vi "ExSimpleAsyncExample.vi"() -> ()   [LabVIEW 2010]
panel:
  in  "Trigger Edge":u32(ring)=1 items=["N/A", "Positive (leading) edge", "Negative (falling) edge"]
  in  "Timing Mode":u32(ring)=1 items=["N/A", "Free Run/Timed", "Trigger First (PM only)", "Ext Sync/Strobed ", "Variable Exp (PM only)", "Flash Mode (PM only)"]
  in  "Temperature":dbl format="%.2f"
  in  "Exposure":dbl min=0.0 step=0.001 format="%.3f"
  in  "stop":bool
  in  "Store":bool
  out "error out":errorcluster
  in  "error in (no error)":errorcluster
  # "ExSimipleAsyncExample:\nThis is a Full Frame Async example. This should work with \nall camera systems. It requires a start for every frame \ncollected. Not all timing modes work for all cameras, also \nthe trigger edge only applies to Princeton Instrument \ncameras. Not all cameras have the ability to set the \ntemperature.\nPressing the stop button stops the example."
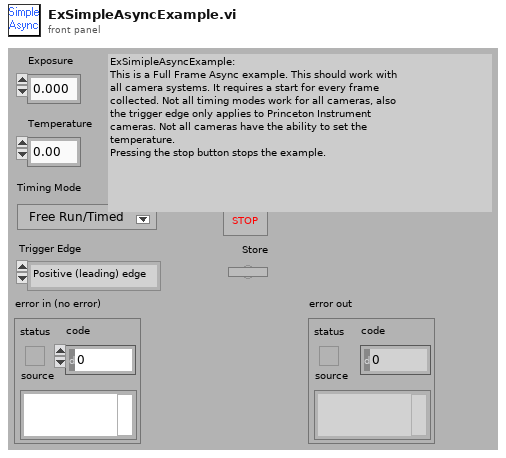
[diagram p1: front panel]
types:
  T1 = cluster{"Acquire mode \n3 is Async":i32, "Exposure":dbl, "Number of Images":i32, "Software Accums":i32}
  T2 = cluster{"Camera Handle":u32, "Pulser Handle":u32, "File Handle":u32, "Display Handle":u32, "Image Handle":u32}
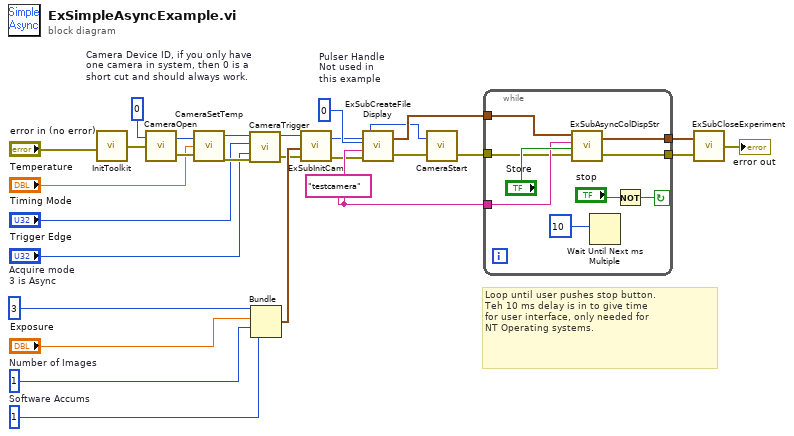
[diagram p0: block diagram]
diagram:
  w10 = 0  # Camera Device ID, if you only have  one camera in system, then 0 is a  short cut and should always work.
  w20 = 0  # Pulser Handle Not used in  this example
  w25 = 1  # Number of Images
  w26 = 3  # Acquire mode  3 is Async
  w24 = 1  # Software Accums
  w27 = "testcamera"
  # "Loop until user pushes stop button.\nTeh 10 ms delay is in to give time \nfor user interface, only needed for \nNT Operating systems."
  n1 = call <userlib>:"InitToolkit.vi"("error in"="error in (no error)") -> ("error out"=w11:errorcluster)
  n2 = call <userlib>:"CameraOpen.vi"("error in"=w11, "Camera Device ID"=w10) -> ("error out"=w8:errorcluster, "Camera Handle"=w9:u32)
  n3 = call <userlib>:"CameraSetTemp.vi"("error in (no error)"=w8, "Temperature"="Temperature", "Camera Handle"=w9) -> ("error out"=w5:errorcluster, "Camera Handle"=w6:u32)
  n4 = call <userlib>:"CameraTrigger.vi"("error in"=w5, "Trigger Edge"="Trigger Edge", "Timing Mode"="Timing Mode", "Camera Handle"=w6) -> ("error out"=w2:errorcluster, "Camera Handle"=w1:u32)
  n5 = Bundle("Acquire mode \n3 is Async"=w26, "Exposure"="Exposure", "Number of Images"=w25, "Software Accums"=w24) -> (w22:T1)  [unwired: 1 in]
  n6 = call "ExSubInitCam.vi"("error in (no error)"=w2, "Camera Information"=w22, "Camera Handle"=w1) -> ("error out"=w21:errorcluster, "Camera Handle"=w16:u32)
  n7 = call "ExSubCreateFileDisplay.vi"("error in (no error)"=w21, "File and Display Name"=w27, "Pulser Handle"=w20, "Camera Handle"=w16) -> ("error out"=w19:errorcluster, "Handles Out"=w18:T2)
  n8 = call <userlib>:"CameraStart.vi"("error in"=w19, "Camera Handle"=w16) -> ("error out"=w17:errorcluster)  [unwired: 1 out]
  n9 = while {
    tunnel: w18 -> [w34]
    tunnel: w17 -> [w32]
    tunnel: w27 -> [w33]
    tunnel: [w30] -> w14
    tunnel: [w31] -> w15
    stop <- w29 continue-if-true
    n10 = call "ExSubAsyncColDispStr.vi"("error in (no error)"=w32, "Store Data"="Store", "Display Title"=w33, "Handle Cluster"=w34) -> ("error out"=w30:errorcluster, "Handle Cluster Out"=w31:T2)
    n11 = Wait Until Next ms Multiple(millisecond multiple=10) -> ()  [unwired: 1 out]
    n12 = Not(x="stop") -> (.not. x?=w29:bool)
  }
  n13 = call "ExSubCloseExperiment.vi"("error in (no error)"=w14, "Handles In"=w15) -> ("error out"=→"error out":errorcluster)
